vi "Sample Out.vi"(8 "error in (no error)":errorcluster, 11 "Storage Line in":refnum<class "Storage Line.lvclass">) -> (0 "error out":errorcluster, 3 "Storage Line out":refnum<class "Storage Line.lvclass">)   [LabVIEW 2015, in "cRIO-Carbondioxide.lvlib" / "CO2-Actor.lvlib" / "Storage Line.lvclass"]
uses:
  Storage Line.lvclass
  Storage Line.lvclass/Storage Line.ctl
  CO2 Actor/CO2 Actor.lvclass
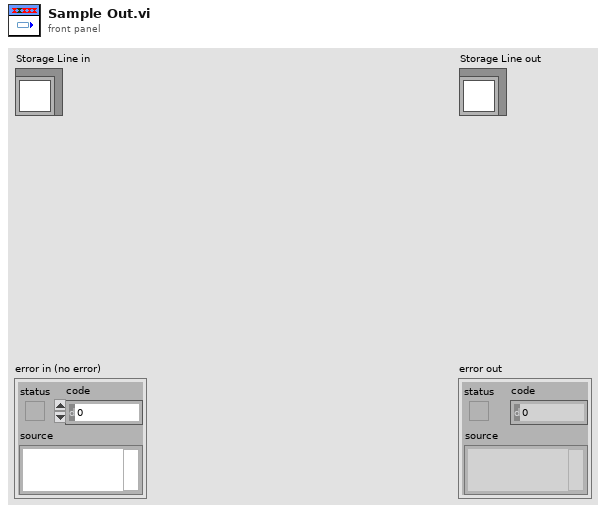
[diagram p1: front panel]
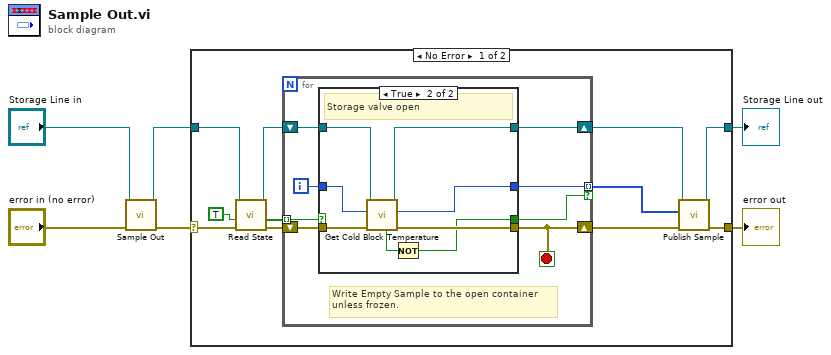
[diagram p0: block diagram]
diagram:
  n1 = call-parent "Sample Out.vi"("error in (no error)"="error in (no error)", "CO2 Actor in"="Storage Line in") -> ("error out"=w4:errorcluster, "CO2 Actor out"=w3:refnum<class "Storage Line.lvclass">)  [unwired: 8 in]
  n2 = case shown="No Error" w4 {
    selector: w4 -> [w16 w38]
    tunnel: w3 -> [w15 w39]
    tunnel: [w7 w39] -> w2
    tunnel: [w10 w38] -> w1
    frame No Error {
      n3 = call "Read State.vi"("error in (no error)"=w16, "Return Boolean Array? (F)"=TRUE, "Storage Line in"=w15) -> ("error out"=w13:errorcluster, "Boolean array"=w12:bool[], "Storage Line out"=w14:refnum<class "Storage Line.lvclass">)  [unwired: 4 in, 2 out]
      n4 = for {
        shift-right: [w23] -> w8
        shift-left: w14 -> [w24]
        shift-right: [w21] -> w11
        shift-left: w13 -> [w25]
        tunnel: w12 -> [w22] mode=indexing
        tunnel: [w19] -> w9 mode=indexing if=w18
        i -> [w20]
        stop <- w21 stop-if-true
        # "Write Empty Sample to the open container\nunless frozen."
        n5 = case shown="True" w22 {
          selector: w22 -> [w27 _]
          tunnel: w25 -> [w28 w37]
          tunnel: [w28 w33] -> w21
          tunnel: w24 -> [w29 w36]
          tunnel: [w29 w34] -> w23
          tunnel: w20 -> [w26 w35]
          tunnel: [w26 w32] -> w19
          tunnel: [w27 w30] -> w18
          frame False {
          }
          frame True {
            # "Storage valve open"
            n6 = call "Get Cold Block Temperature.vi"("error in (no error)"=w37, "Storage Index"=w35, "Storage Line in"=w36) -> ("error out"=w33:errorcluster, "Storage Index"=w32:i32, "Storage Line out"=w34:refnum<class "Storage Line.lvclass">, "Frozen?"=w31:bool)  [unwired: 4 in, 1 out]
            n7 = Not(x=w31) -> (.not. x?=w30:bool)
          }
        }
      }
      n8 = call "Publish Sample.vi"("error in (no error)"=w11, "Indice"=w9, "Storage Line in"=w8) -> ("error out"=w10:errorcluster, "Storage Line out"=w7:refnum<class "Storage Line.lvclass">)  [unwired: 7 in]
    }
    frame Error {
    }
  }
  "error out" <- w1
  "Storage Line out" <- w2
